vi "test-median-filter.vi"() -> ()   [LabVIEW 2019]
uses:
  <vilib>/Rock Robotics/WPI/ThirdParty/JAS_Junk/TrajLib/MEDIAN_FILTER.ctl
  <vilib>/Rock Robotics/WPI/ThirdParty/JAS_Junk/TrajLib/Trajectory_Library.lvlib
panel:
  out "MedianValue 6 = 3.5":dbl
  out "MedianValue 5 = 3":dbl
  out "MedianValue 4 = 1.5":dbl
  out "MedianValue  3  = 0":dbl
  out "MedianValue 2 = 1.5":dbl
  out "MedianValue   1 = 3":dbl
  out "Out MEDIAN_FILTER 2":T1 {"ValueBuffer" format="%13.5g"}
  out "T3--X--Value":dbl
  out "T3 -- X -- 0":dbl
  out "Out MEDIAN_FILTER":T1 {"ValueBuffer" format="%13.5g"}
  out "T2--X--Value":dbl
  out "T0--X--Value":dbl
  out "T2 -- X -- 0":dbl
  out "T1 -- X -- 0":dbl
  out "T0 -- X -- 0":dbl
  # "Median Filter Test"
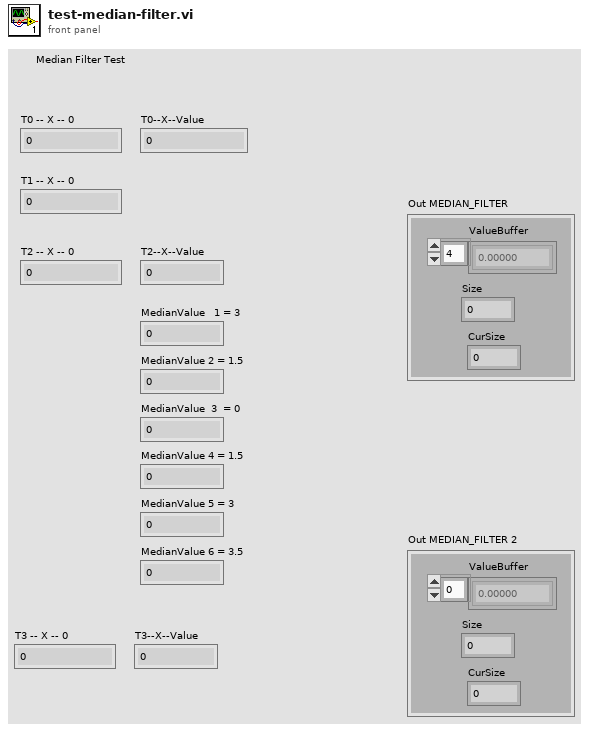
[diagram p1: front panel]
types:
  T1 = typedef "Trajectory_Library.lvlib/MEDIAN_FILTER.ctl" = cluster{"ValueBuffer":dbl[], "Size":i32, "CurSize":i32}
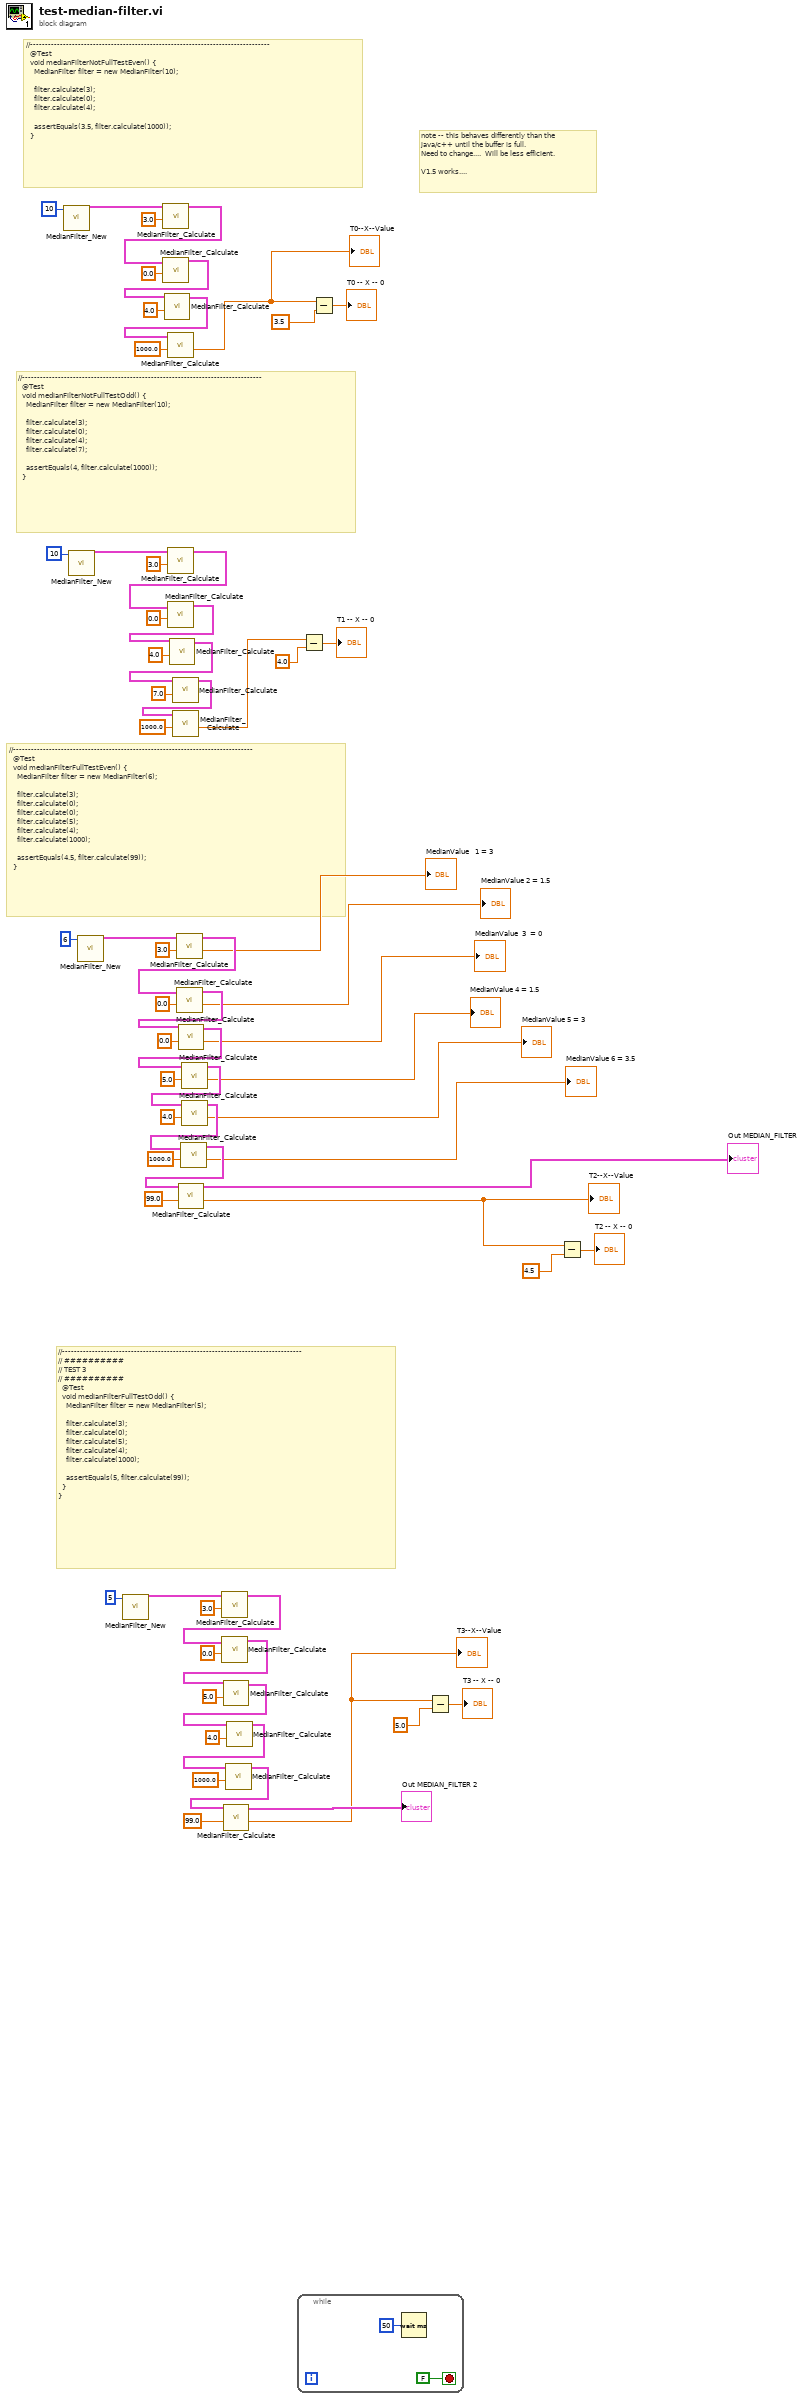
[diagram p0: block diagram]
diagram:
  # "//--------------------------------------------------------------------------------\n// ##########\n// TEST 3\n// ##########\n  @Test\n  void medianFilterFullTestOdd() {\n    MedianFilter filter = new MedianFilter(5);\n\n    filter.calculate(3);\n    filter.calculate(0);\n    filter.calculate(5);\n    filter.calculate(4);\n    filter.calculate(1000);\n\n    assertEquals(5, filter.calculate(99));\n  }\n}"
  # "note -- this behaves differently than the \njava/c++ until the buffer is full.\nNeed to change....  Will be less efficient.\n\nV1.5 works...."
  # "//--------------------------------------------------------------------------------\n  @Test\n  void medianFilterFullTestEven() {\n    MedianFilter filter = new MedianFilter(6);\n\n    filter.calculate(3);\n    filter.calculate(0);\n    filter.calculate(0);\n    filter.calculate(5);\n    filter.calculate(4);\n    filter.calculate(1000);\n\n    assertEquals(4.5, filter.calculate(99));\n  }"
  # "//--------------------------------------------------------------------------------\n  @Test\n  void medianFilterNotFullTestOdd() {\n    MedianFilter filter = new MedianFilter(10);\n\n    filter.calculate(3);\n    filter.calculate(0);\n    filter.calculate(4);\n    filter.calculate(7);\n\n    assertEquals(4, filter.calculate(1000));\n  }"
  # "//--------------------------------------------------------------------------------\n  @Test\n  void medianFilterNotFullTestEven() {\n    MedianFilter filter = new MedianFilter(10);\n\n    filter.calculate(3);\n    filter.calculate(0);\n    filter.calculate(4);\n\n    assertEquals(3.5, filter.calculate(1000));\n  }"
  n1 = call <vilib>:"MedianFilter_New.vi"("Samples"=10) -> ("MEDIAN_FILTER"=w58:T1)  [unwired: 10 in]
  n2 = call <vilib>:"MedianFilter_New.vi"("Samples"=10) -> ("MEDIAN_FILTER"=w49:T1)  [unwired: 10 in]
  n3 = call <vilib>:"MedianFilter_New.vi"("Samples"=6) -> ("MEDIAN_FILTER"=w36:T1)  [unwired: 10 in]
  n4 = call <vilib>:"MedianFilter_New.vi"("Samples"=5) -> ("MEDIAN_FILTER"=w19:T1)  [unwired: 10 in]
  n5 = call <vilib>:"MedianFilter_Calculate.vi"("Input Value"=3.0, "In MEDIAN_FILTER"=w58) -> ("Out MEDIAN_FILTER"=w57:T1)  [unwired: 8 in, 1 out]
  n6 = call <vilib>:"MedianFilter_Calculate.vi"("Input Value"=0.0, "In MEDIAN_FILTER"=w57) -> ("Out MEDIAN_FILTER"=w56:T1)  [unwired: 8 in, 1 out]
  n7 = call <vilib>:"MedianFilter_Calculate.vi"("Input Value"=4.0, "In MEDIAN_FILTER"=w56) -> ("Out MEDIAN_FILTER"=w55:T1)  [unwired: 8 in, 1 out]
  n8 = call <vilib>:"MedianFilter_Calculate.vi"("Input Value"=1000.0, "In MEDIAN_FILTER"=w55) -> ("MedianValue"=w63:dbl)  [unwired: 8 in, 1 out]
  "T0--X--Value" <- w63
  n9 = call <vilib>:"MedianFilter_Calculate.vi"("Input Value"=3.0, "In MEDIAN_FILTER"=w49) -> ("Out MEDIAN_FILTER"=w48:T1)  [unwired: 8 in, 1 out]
  n10 = call <vilib>:"MedianFilter_Calculate.vi"("Input Value"=0.0, "In MEDIAN_FILTER"=w48) -> ("Out MEDIAN_FILTER"=w47:T1)  [unwired: 8 in, 1 out]
  n11 = call <vilib>:"MedianFilter_Calculate.vi"("Input Value"=4.0, "In MEDIAN_FILTER"=w47) -> ("Out MEDIAN_FILTER"=w46:T1)  [unwired: 8 in, 1 out]
  n12 = call <vilib>:"MedianFilter_Calculate.vi"("Input Value"=7.0, "In MEDIAN_FILTER"=w46) -> ("Out MEDIAN_FILTER"=w44:T1)  [unwired: 8 in, 1 out]
  n13 = call <vilib>:"MedianFilter_Calculate.vi"("Input Value"=1000.0, "In MEDIAN_FILTER"=w44) -> ("MedianValue"=w42:dbl)  [unwired: 8 in, 1 out]
  n14 = call <vilib>:"MedianFilter_Calculate.vi"("Input Value"=3.0, "In MEDIAN_FILTER"=w36) -> ("MedianValue"=→"MedianValue   1 = 3":dbl, "Out MEDIAN_FILTER"=w35:T1)  [unwired: 8 in]
  n15 = call <vilib>:"MedianFilter_Calculate.vi"("Input Value"=0.0, "In MEDIAN_FILTER"=w35) -> ("MedianValue"=→"MedianValue 2 = 1.5":dbl, "Out MEDIAN_FILTER"=w34:T1)  [unwired: 8 in]
  n16 = call <vilib>:"MedianFilter_Calculate.vi"("Input Value"=0.0, "In MEDIAN_FILTER"=w34) -> ("MedianValue"=→"MedianValue  3  = 0":dbl, "Out MEDIAN_FILTER"=w33:T1)  [unwired: 8 in]
  n17 = call <vilib>:"MedianFilter_Calculate.vi"("Input Value"=5.0, "In MEDIAN_FILTER"=w33) -> ("MedianValue"=→"MedianValue 4 = 1.5":dbl, "Out MEDIAN_FILTER"=w31:T1)  [unwired: 8 in]
  n18 = call <vilib>:"MedianFilter_Calculate.vi"("Input Value"=4.0, "In MEDIAN_FILTER"=w31) -> ("MedianValue"=→"MedianValue 5 = 3":dbl, "Out MEDIAN_FILTER"=w29:T1)  [unwired: 8 in]
  n19 = call <vilib>:"MedianFilter_Calculate.vi"("Input Value"=1000.0, "In MEDIAN_FILTER"=w29) -> ("MedianValue"=→"MedianValue 6 = 3.5":dbl, "Out MEDIAN_FILTER"=w27:T1)  [unwired: 8 in]
  n20 = call <vilib>:"MedianFilter_Calculate.vi"("Input Value"=99.0, "In MEDIAN_FILTER"=w27) -> ("MedianValue"=w3:dbl, "Out MEDIAN_FILTER"=→"Out MEDIAN_FILTER":T1)  [unwired: 8 in]
  "T2--X--Value" <- w3
  n21 = call <vilib>:"MedianFilter_Calculate.vi"("Input Value"=3.0, "In MEDIAN_FILTER"=w19) -> ("Out MEDIAN_FILTER"=w18:T1)  [unwired: 8 in, 1 out]
  n22 = call <vilib>:"MedianFilter_Calculate.vi"("Input Value"=0.0, "In MEDIAN_FILTER"=w18) -> ("Out MEDIAN_FILTER"=w17:T1)  [unwired: 8 in, 1 out]
  n23 = call <vilib>:"MedianFilter_Calculate.vi"("Input Value"=5.0, "In MEDIAN_FILTER"=w17) -> ("Out MEDIAN_FILTER"=w16:T1)  [unwired: 8 in, 1 out]
  n24 = call <vilib>:"MedianFilter_Calculate.vi"("Input Value"=4.0, "In MEDIAN_FILTER"=w16) -> ("Out MEDIAN_FILTER"=w11:T1)  [unwired: 8 in, 1 out]
  n25 = call <vilib>:"MedianFilter_Calculate.vi"("Input Value"=1000.0, "In MEDIAN_FILTER"=w11) -> ("Out MEDIAN_FILTER"=w13:T1)  [unwired: 8 in, 1 out]
  n26 = call <vilib>:"MedianFilter_Calculate.vi"("Input Value"=99.0, "In MEDIAN_FILTER"=w13) -> ("MedianValue"=w2:dbl, "Out MEDIAN_FILTER"=→"Out MEDIAN_FILTER 2":T1)  [unwired: 8 in]
  "T3--X--Value" <- w2
  n27 = while {
    stop <- FALSE stop-if-true
    n28 = Wait (ms)(milliseconds to wait=u32 50) -> ()  [unwired: 1 out]
  }
  n29 = Subtract(x=w42, y=4.0) -> (x-y=→"T1 -- X -- 0":dbl)
  n30 = Subtract(x=w63, y=3.5) -> (x-y=→"T0 -- X -- 0":dbl)
  n31 = Subtract(x=w2, y=5.0) -> (x-y=→"T3 -- X -- 0":dbl)
  n32 = Subtract(x=w3, y=4.5) -> (x-y=→"T2 -- X -- 0":dbl)
